vi "Untitled 1.vi"() -> ()   [LabVIEW 2016]
uses:
  Classes/Controller/I-O/NI-DAQ Folder/NI-DAQ.lvclass
panel:
  in  "Value":bool=TRUE
  in  "Channel":i32
  in  "stop":bool
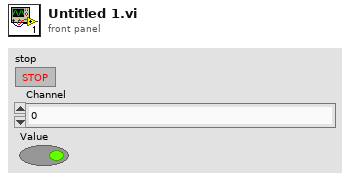
[diagram p1: front panel]
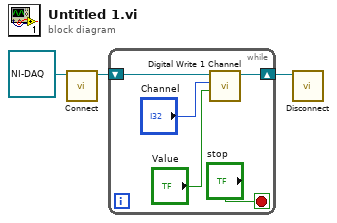
[diagram p0: block diagram]
diagram:
  n1 = call-dynamic "Connect.vi"("NI-DAQ in"=refnum<class "NI-DAQ.lvclass"> refnum ("NI-DAQ.lvclass")) -> ("NI-DAQ out"=w2:refnum<class "NI-DAQ.lvclass">)  [unwired: 9 in, 1 out]
  n2 = while {
    shift-right: [w7] -> w1
    shift-left: w2 -> [w8]
    stop <- "stop" stop-if-true
    n3 = call-dynamic "Digital Write 1 Channel.vi"("Value"="Value", "Channel"="Channel", "NI-DAQ.lvclass"=w8) -> ("NI-DAQ.lvclass 2"=w7:refnum<class "NI-DAQ.lvclass">)  [unwired: 7 in, 1 out]
  }
  n4 = call-dynamic "Disconnect.vi"("I-O in"=w1) -> ()  [unwired: 9 in, 1 out]
